vi "Read status mMc Edited.vi"(1 "Port":T1={"P type"=0, "reference"="", " Terminator "="\r\n", "Timeout"=300} {"Timeout" step=10; "P type" items=["none", "RS-232C"]}, 3 "error in (no error)":errorcluster, 5 "Controller #":string) -> (6 "Moving?":bool, 7 "In position?":bool, 9 "error out":errorcluster)   [LabVIEW 2021]
panel:
  out "status array":bool[](array[boolean])
  # "Read status"
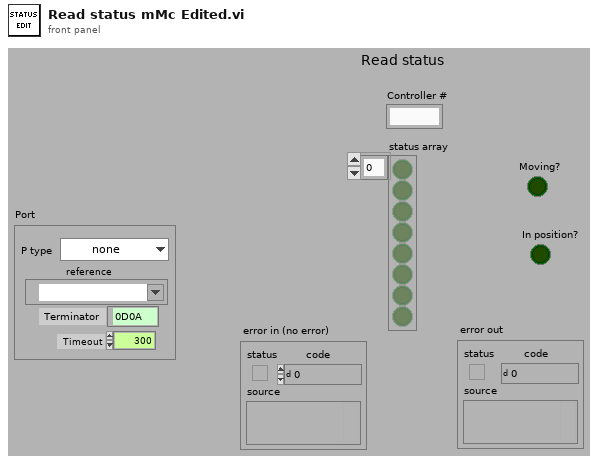
[diagram p1: front panel]
types:
  T1 = cluster{"P type":u16, "reference":refnum<visa-resource-name>, " Terminator ":string, "Timeout":i32}
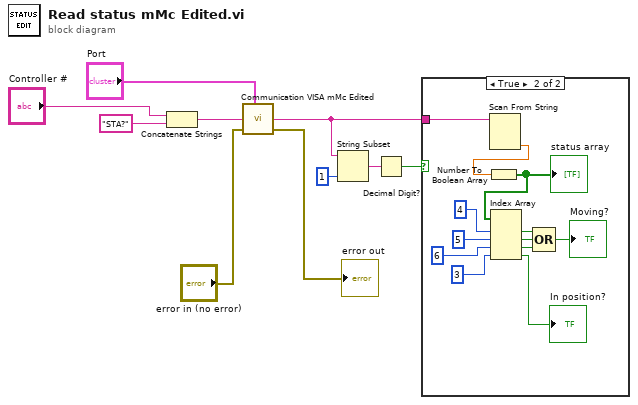
[diagram p0: block diagram]
diagram:
  n1 = Concatenate Strings("Controller #", "STA?") -> (w6:string)
  n2 = call "Communication VISA mMc Edited.vi"("Port"="Port", "Command"=w6, "error in (no error)"="error in (no error)") -> ("Return"=w1:string, "error out"=→"error out":errorcluster)  [unwired: 3 in, 2 out]
  n3 = String Subset(string=w1, length (rest)=1 ("length (rest)")) -> (substring=w3:string)  [unwired: 1 in]
  n4 = Decimal Digit?(1:w3) -> (0:w2:bool)
  n5 = case shown="True" w2 {
    tunnel: w1 -> [_ w22]
    frame False {
    }
    frame True {
      n6 = Scan From String(input string=w22) -> (output 1=w21:dbl)  [unwired: 4 in, 3 out]
      n7 = Number To Boolean Array(number=w21) -> (Boolean array=w20:bool[])
      "status array" <- w20
      n8 = Index Array(array=w20, index #1=4 ("index"), index #2=5 ("index"), index #3=6 ("index"), index #4=3 ("index")) -> (element #1=w16:bool, element #2=w15:bool, element #3=w14:bool, element #4=→"In position?":bool)
      n9 = Compound Arithmetic op=OR(w16, w15, w14) -> (→"Moving?":bool)
    }
  }
